vi "Current Limit.vi"(8 "Scale Min":dbl, 9 "Slider Value":dbl(knob) scale=-50.0..50.0, 11 "Scale Max":dbl) -> (2 "Fill Color":u32)   [LabVIEW 2022 SP3]
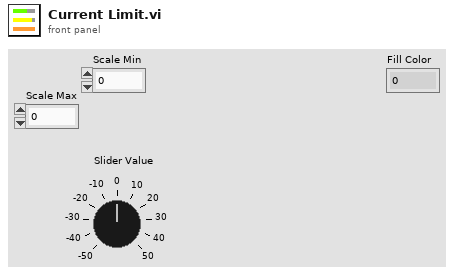
[diagram p1: front panel]
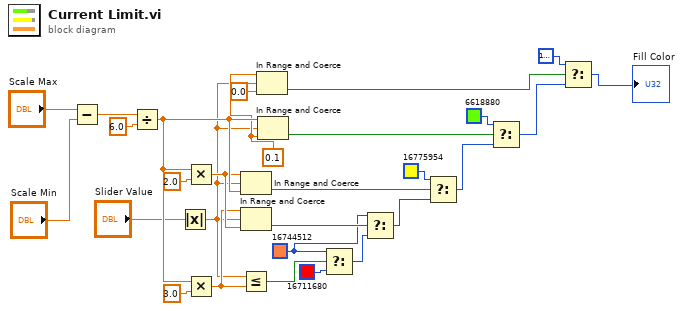
[diagram p0: block diagram]
diagram:
  w11 = u32 16744512 ("Fill Color")
  w6 = 0.1 ("lower limit")
  n1 = Subtract(x="Scale Max", y="Scale Min") -> (x-y=w27:dbl)
  n2 = Divide(x=w27, y=6.0) -> (x/y=w23:dbl)
  n3 = Absolute Value(x="Slider Value") -> (abs(x)=w5:dbl)
  n4 = Multiply(x=w23, y=2.0) -> (x*y=w19:dbl)
  n5 = Multiply(x=w23, y=3.0) -> (x*y=w18:dbl)
  n6 = In Range and Coerce(upper limit=w19, x=w5, lower limit=w23) -> (In Range?=w22:bool)  [unwired: 1 out]
  n7 = In Range and Coerce(upper limit=w18, x=w5, lower limit=w19) -> (In Range?=w21:bool)  [unwired: 1 out]
  n8 = Less Or Equal?(x=w5, y=w18) -> (x <= y?=w17:bool)
  n9 = In Range and Coerce(upper limit=w6, x=w5, lower limit=0.0) -> (In Range?=w1:bool)  [unwired: 1 out]
  n10 = In Range and Coerce(upper limit=w23, x=w5, lower limit=w6) -> (In Range?=w24:bool)  [unwired: 1 out]
  n11 = Select(t=w11, s=w17, f=u32 16711680 ("Fill Color")) -> (s? t:f=w15:u32)
  n12 = Select(t=w11, s=w21, f=w15) -> (s? t:f=w20:u32)
  n13 = Select(t=u32 16775954 ("Fill Color"), s=w22, f=w20) -> (s? t:f=w13:u32)
  n14 = Select(t=u32 6618880 ("Fill Color"), s=w24, f=w13) -> (s? t:f=w2:u32)
  n15 = Select(t=u32 16777216 ("Fill Color"), s=w1, f=w2) -> (s? t:f=→"Fill Color":u32)
